vi "Example_Get Instrument ID.vi"() -> ()   [LabVIEW 2011]
panel:
  in  "Ethernet":T1={"Port"=10001, "Timeout"=1000, "IP Address"=""}
  in  "Remote Mode":u16(ring) items=["USB", "RS232", "GPIB", "Ethernet"]
  in  "Baud Rate (921600)":u32=921600
  out "Read Buffer":string
  out "Error out":errorcluster caption="error out"
  in  "error in (no error)":errorcluster
  in  "VISA resource name":refnum<visa-resource-name>
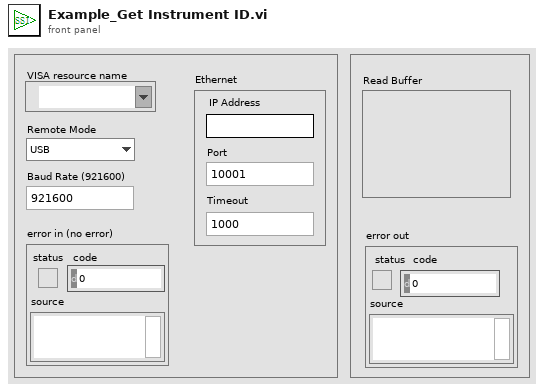
[diagram p1: front panel]
types:
  T1 = cluster{"Port":u32, "Timeout":u32, "IP Address":string}
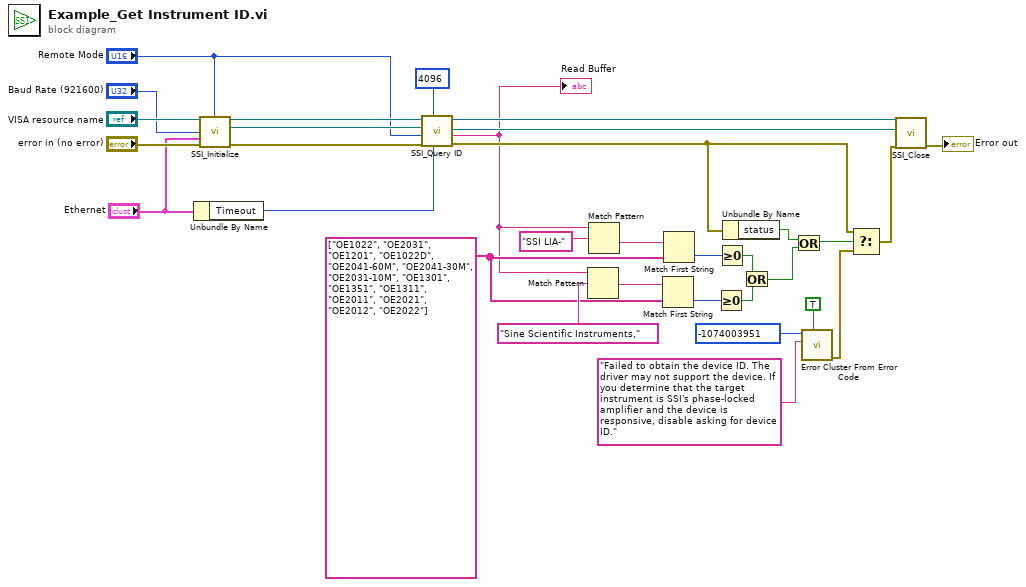
[diagram p0: block diagram]
diagram:
  w3 = string[] ["OE1022", "OE2031", "OE1201", "OE1022D", "OE2041-60M", "OE2041-30M", "OE2031-10M", "OE1301", "OE1351", "OE1311", "OE2011", "OE2021", "OE2012", "OE2022"] ("string array")
  n1 = Unbundle By Name("Ethernet") -> ("Timeout"=w12:u32)
  n2 = call "SSI_Initialize.vi"("VISA resource name"="VISA resource name", "Remote Mode"="Remote Mode", "baud rate (921600)"="Baud Rate (921600)", "Ethernet"="Ethernet", "error in (no error)"="error in (no error)") -> ("VISA resource name out"=w22:refnum<visa-resource-name>, "connection ID(Ethernet)"=w20:refnum<k5>, "error out"=w21:errorcluster)  [unwired: 8 in]
  n3 = call "SSI_Query ID.vi"("Timeout"=w12, "Number of bytes"=u32 4096, "Error in (no error)"=w21, "Remote Mode"="Remote Mode", "Connection ID in"=w20, "VISA resource name"=w22) -> ("Error out"=w16:errorcluster, "Read Buffer"=w2:string, "Connection ID out"=w18:refnum<k5>, "VISA resource  out"=w19:refnum<visa-resource-name>)  [unwired: 2 in]
  "Read Buffer" <- w2
  n4 = Match Pattern(string=w2, regular expression="Sine Scientific Instruments," ("字符串")) -> (after substring=w6:string)  [unwired: 1 in, 3 out]
  n5 = Match Pattern(string=w2, regular expression="SSI LIA-" ("正则表达式")) -> (after substring=w10:string)  [unwired: 1 in, 3 out]
  n6 = Match First String(2:w3, 3:w6) -> (0:w8:i32)  [unwired: 1 out]
  n7 = Match First String(2:w3, 3:w10) -> (0:w11:i32)  [unwired: 1 out]
  n8 = Greater Or Equal To 0?(x=w8) -> (x >= 0?=w5:bool)
  n9 = Greater Or Equal To 0?(x=w11) -> (x >= 0?=w9:bool)
  n10 = Unbundle By Name(w16) -> ("status"=w17:bool)
  n11 = Or(x=w9, y=w5) -> (x .or. y?=w4:bool)
  n12 = Or(x=w17, y=w4) -> (x .or. y?=w30:bool)
  n13 = call <vilib>:"Error Cluster From Error Code.vi"("show call chain? (False)"=TRUE, "error message (\"\")"="Failed to obtain the device ID. The driver may not support the device. If you determine that the target instrument is SSI's phase-locked amplifier and the device is responsive, disable asking for device ID." ("Source (VI Name)"), "error code (0)"=-1074003951 ("Code")) -> ("error out"=w26:errorcluster)  [unwired: 1 in, 5 out]
  n14 = Select(t=w16, s=w30, f=w26) -> (s? t:f=w23:errorcluster)
  n15 = call "SSI_Close.vi"("Error in (no error)"=w23, "Connection ID in"=w18, "VISA resource name"=w19) -> ("Error out"=→"Error out":errorcluster)  [unwired: 4 in]
